vi "Get Default Object.vi"() -> (1 "Object Dictionary":refnum<class "objdict.lvclass">)   [LabVIEW 2015, in "objdict.lvclass"]
doc: "Returns the default instance of <b>objdict.lvclass</b>. It is safer to use this VI than a constant of the class because this VI initializes all properties of the class explicitly, guaranteeing the default values intended by the class design."
uses:
  objdict.lvclass
  objdict.lvclass/objdict.ctl
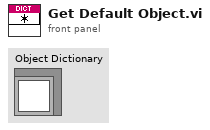
[diagram p1: front panel]
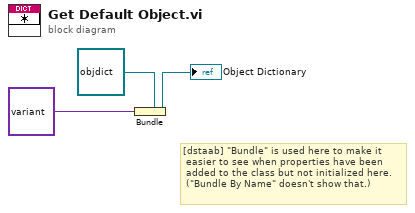
[diagram p0: block diagram]
diagram:
  # "[dstaab] \"Bundle\" is used here to make it\n easier to see when properties have been\n added to the class but not initialized here.\n (\"Bundle By Name\" doesn't show that.)"
  n1 = Bundle(cluster=refnum<class "objdict.lvclass"> refnum ("Object LUT"), variant ("dict")) -> (→"Object Dictionary":refnum<class "objdict.lvclass">)
